vi "BASE-Main.vi"() -> ()   [LabVIEW 2017]
uses:
  <vilib>/Utility/error.llb/DialogType.ctl
  55ed0eea-cd20-493f-8468-85b8c1a0a0c0.vi
panel:
  out "Status Number":i32
  out "Status":i32(ring)=1 items=["Stopped"=1, "StartPending"=2, "StopPending"=3, "Running"=4, "ContinuePending"=5, "PausePending"=6, "Paused"=7]
  in  "Modify SN":bool
  in  "PRINT":bool
  in  "Torque IO Status":bool
  in  "Ass IO Status":bool
  in  "Recipe":bool
  out "error out":errorcluster
  in  "Logout":bool
  in  "Stop":bool
  in  "Create Login":bool
  in  "Reports":bool
  in  "Start":bool
  out "Time":string
  out "Date":string
  in  "Login":bool
  # "KAPSE SONS ROBOTICS\n& AUTOMATION"
  # "RBC ORVM"
types:
  T1 = typedef "DialogType.ctl" = u16
  T2 = enum32{"Invalid", "Standard", "Closed", "Hidden", "Minimized", "Maximized"}
  T3 = enum8{"Enabled", "Disabled", "Disabled and Grayed Out"}
  T4 = enum32{"invalid app kind", "Development System", "Run Time System", "Student Edition", "Embedded LabVIEW", "Evaluation", "Custom"}
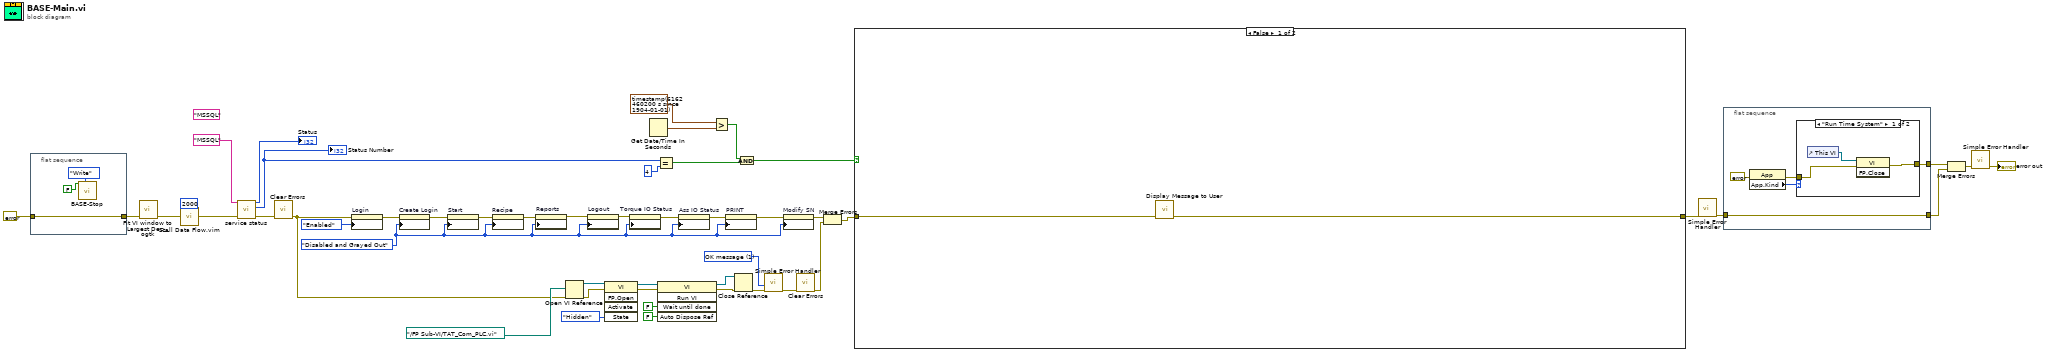
[diagram p0: block diagram]
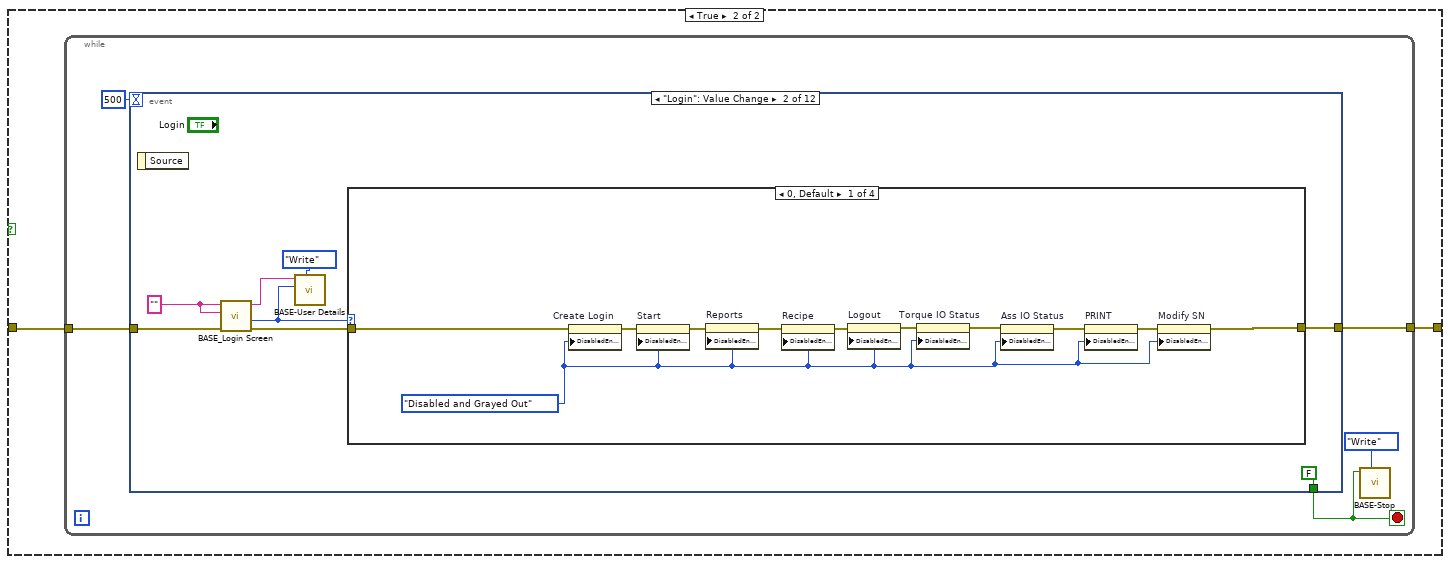
[diagram p3: hidden frame]
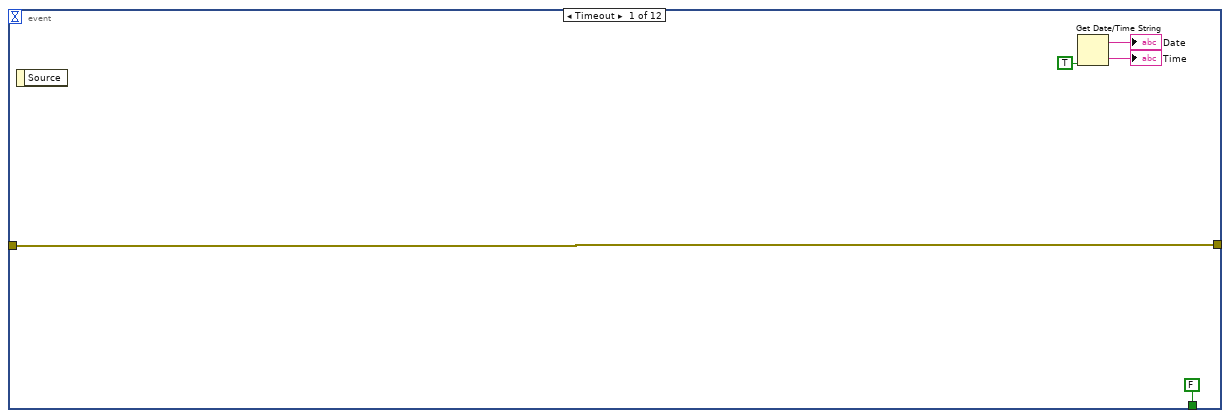
[diagram p4: hidden frame]
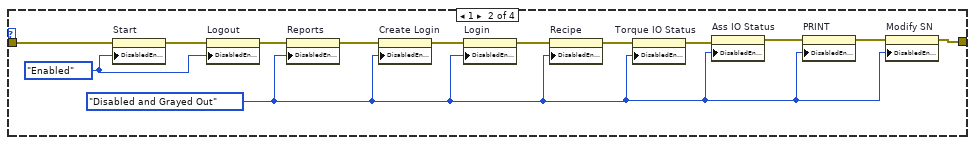
[diagram p5: hidden frame]
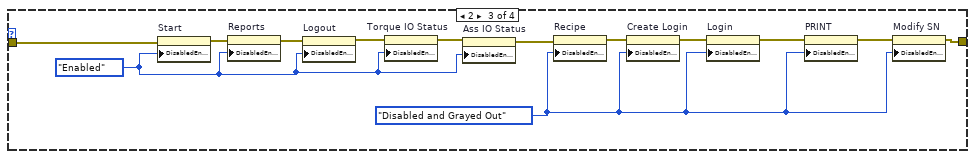
[diagram p6: hidden frame]
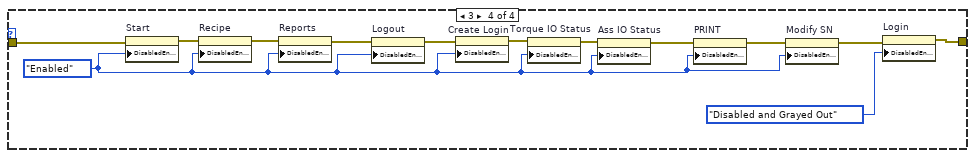
[diagram p7: hidden frame]
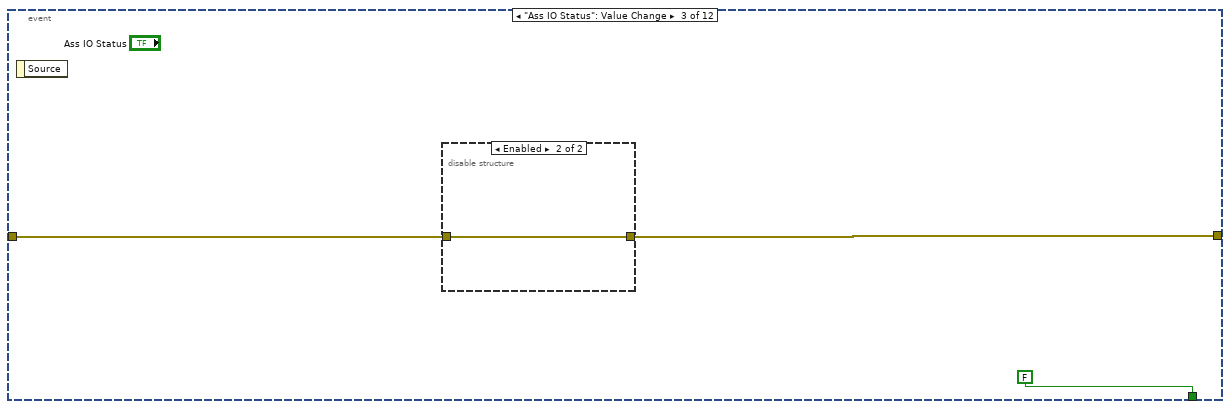
[diagram p8: hidden frame]
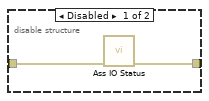
[diagram p9: hidden frame]
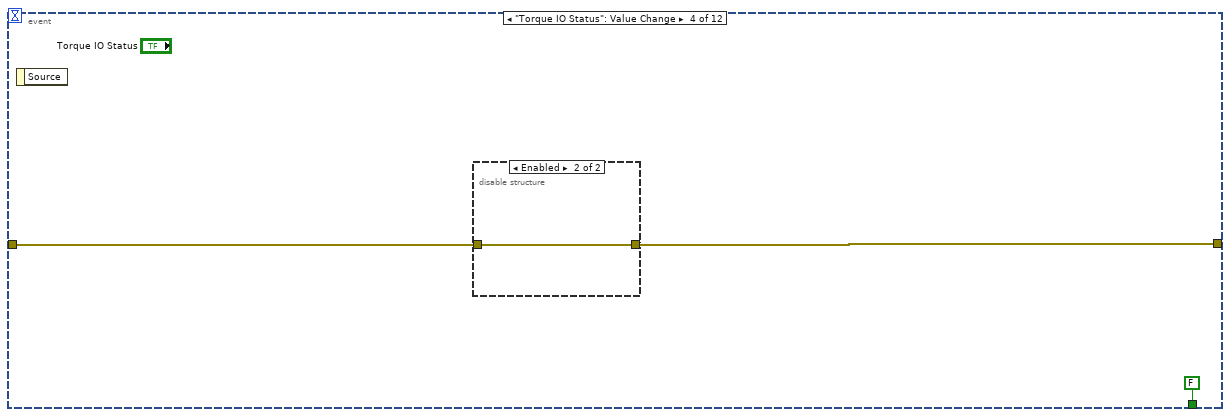
[diagram p10: hidden frame]
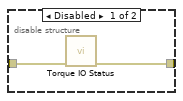
[diagram p11: hidden frame]
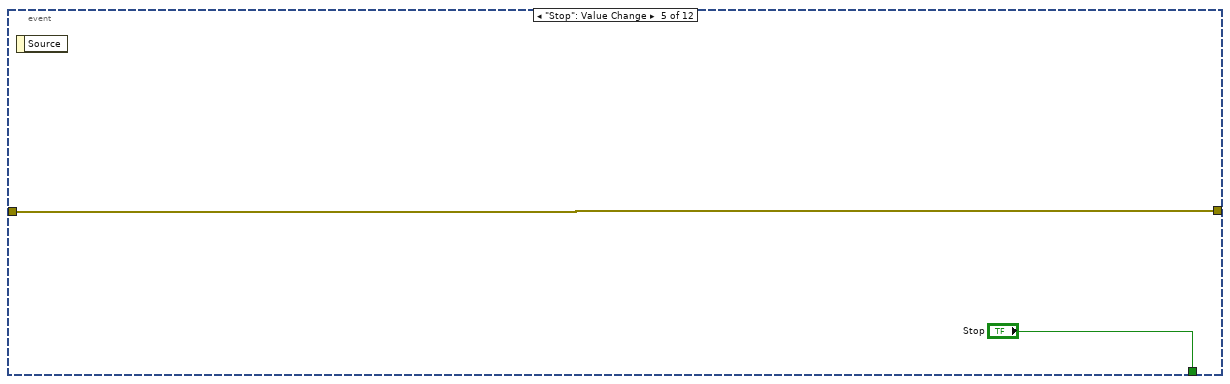
[diagram p12: hidden frame]
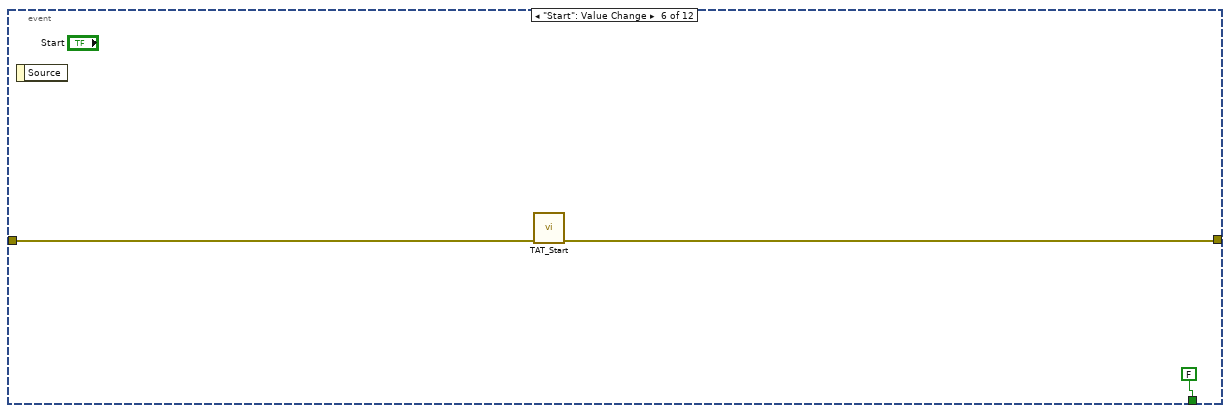
[diagram p13: hidden frame]
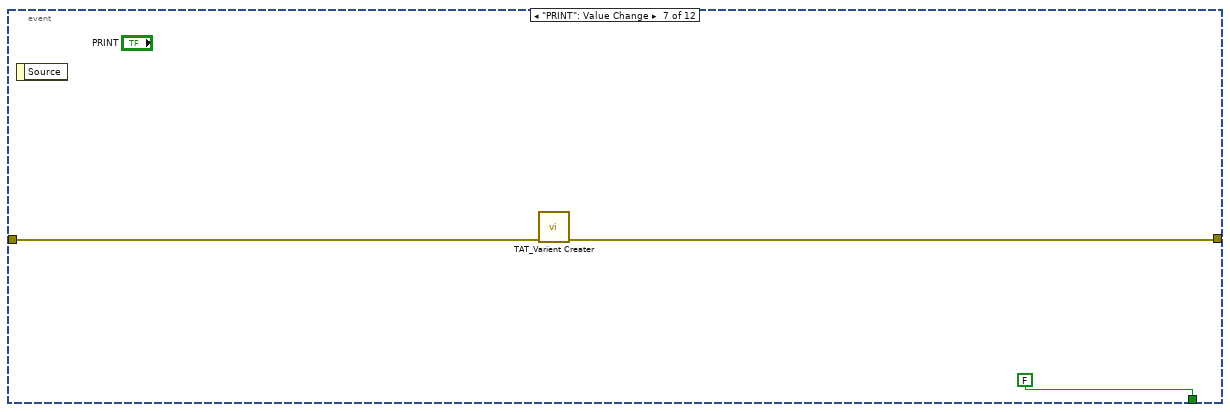
[diagram p14: hidden frame]
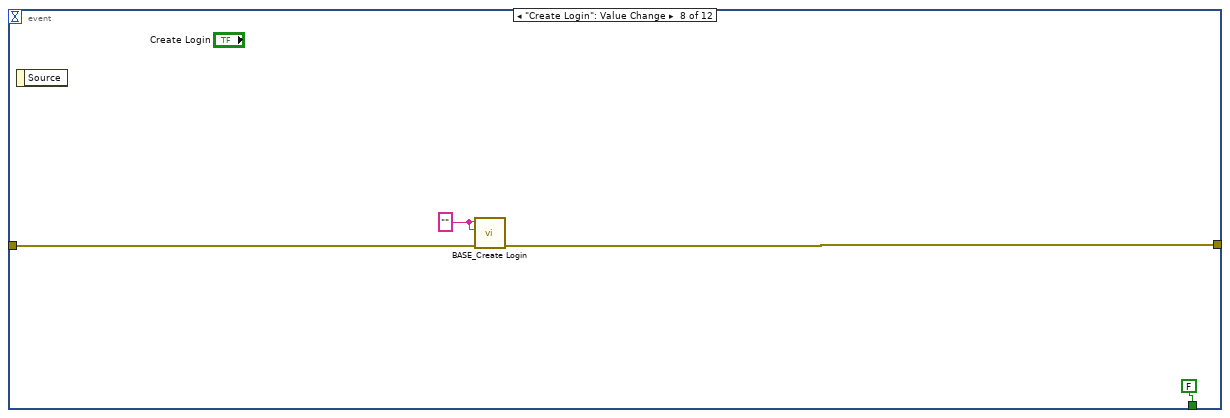
[diagram p15: hidden frame]
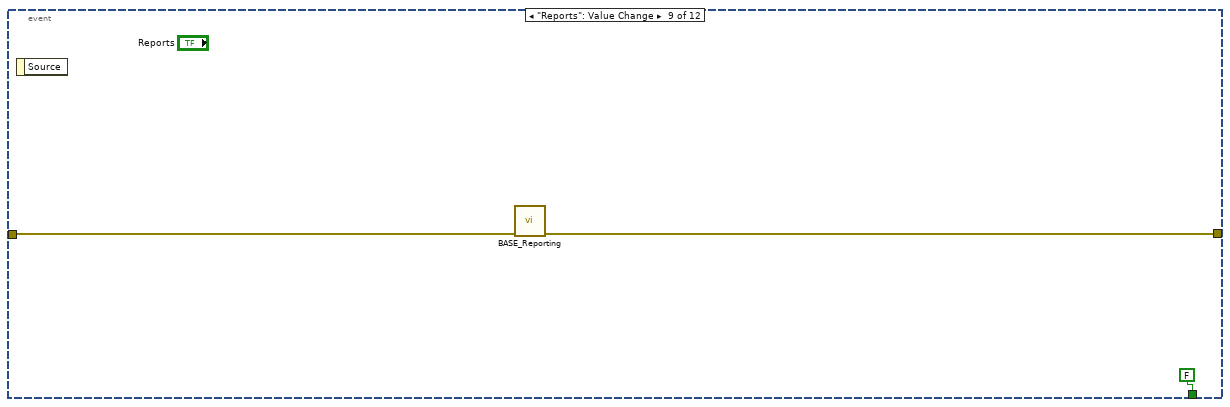
[diagram p16: hidden frame]
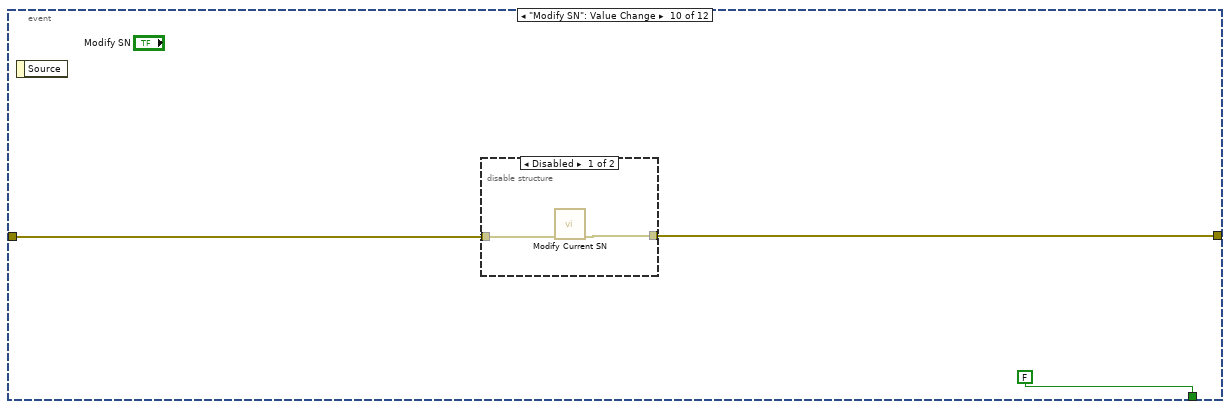
[diagram p17: hidden frame]
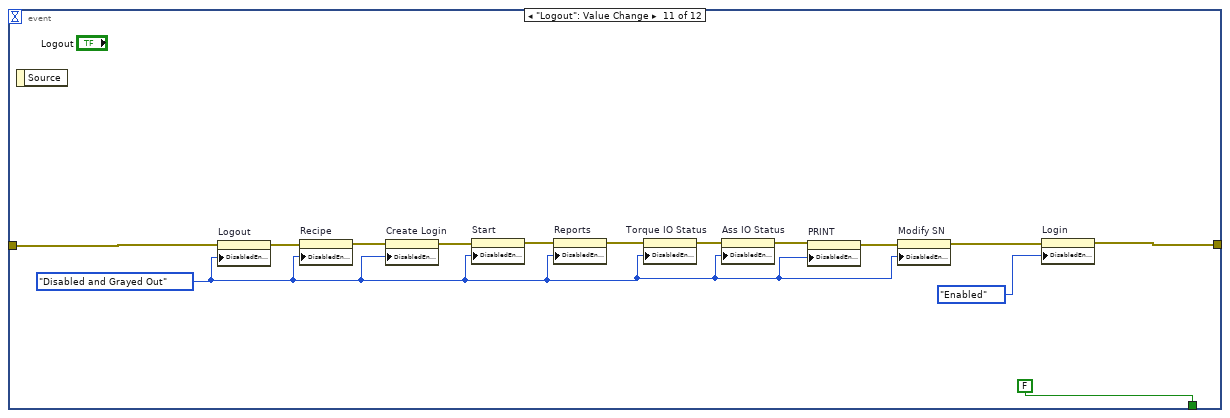
[diagram p19: hidden frame]
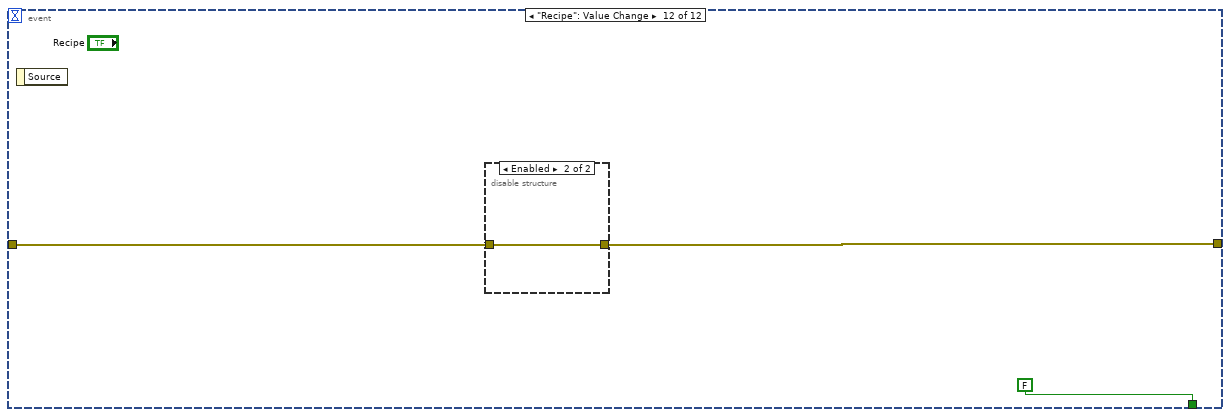
[diagram p20: hidden frame]
diagram:
  (unwired) "MSSQL" ("Service Name")
  w18 = T1 1 items=["no dialog", "OK message", "continue or stop message", "OK message + warnings", "continue/stop + warnings"] ("type of dialog (OK msg:1)")
  w33 = T3."Disabled and Grayed Out" ("Disabled")
  n1 = flat-sequence {
    tunnel: [w52] -> w32
    tunnel: errorcluster {"status"=FALSE, "code"=0, "source"=""} ("error constant") -> [w52]
    frame #0 {
      n2 = call "BASE-Stop.vi"("Enum"=enum16{"Read", "Write"}."Write", "Stop"=FALSE) -> ()  [unwired: 9 in, 1 out]
    }
  }
  n3 = call <userlib>:"Fit VI window to Largest Dec__ogtk.vi"("error in (no error)"=w32) -> ("error out"=w3:errorcluster)  [unwired: 5 in, 1 out]
  n4 = call "Stall Data Flow.vim"("value in"=w3, "milliseconds to wait"=u32 2000) -> ("value out"=w2:errorcluster)  [unwired: 1 out]
  n5 = call "service status.vi"("error in"=w2, "Service Name"="MSSQL") -> ("error out"=w10:errorcluster, "Status Number"=w12:i32, "Status"=→"Status":i32)  [unwired: 6 in, 1 out]
  "Status Number" <- w12
  n6 = call <vilib>:"Clear Errors.vi"("error in (no error)"=w10) -> ("error out"=w9:errorcluster)  [unwired: 5 in, 1 out]
  n7 = property on="Login" class="Bool"(error in=w9, "DisabledEnum"=T3."Enabled" ("Disabled")) -> (error out=w43:errorcluster)  [unwired: 1 in, 1 out]
  n8 = property on="Create Login" class="Bool"(error in=w43, "DisabledEnum"=w33) -> (error out=w48:errorcluster)  [unwired: 1 in, 1 out]
  n9 = property on="Start" class="Bool"(error in=w48, "DisabledEnum"=w33) -> (error out=w39:errorcluster)  [unwired: 1 in, 1 out]
  n10 = property on="Recipe" class="Bool"(error in=w39, "DisabledEnum"=w33) -> (error out=w38:errorcluster)  [unwired: 1 in, 1 out]
  n11 = property on="Reports" class="Bool"(error in=w38, "DisabledEnum"=w33) -> (error out=w41:errorcluster)  [unwired: 1 in, 1 out]
  n12 = Open VI Reference(vi path=path "../FP Sub-VI/TAT_Com_PLC.vi", error in (no error)=w9) -> (vi reference=w28:refnum<vi>, error out=w29:errorcluster)  [unwired: 4 in]
  n13 = property on="Logout" class="Bool"(error in=w41, "DisabledEnum"=w33) -> (error out=w37:errorcluster)  [unwired: 1 in, 1 out]
  n14 = invoke class="VI" method="FP.Open"(reference=w28, error in=w29, "State"=T2."Hidden") -> (reference out=w31:refnum<vi>, error out=w30:errorcluster)  [unwired: 2 in, 3 out]
  n15 = property on="Torque IO Status" class="Bool"(error in=w37, "DisabledEnum"=w33) -> (error out=w36:errorcluster)  [unwired: 1 in, 1 out]
  n16 = Get Date/Time In Seconds() -> (seconds since 1Jan1904=w5:timestamp)
  n17 = Equal?(x=w12, y=4) -> (x = y?=w8:bool)
  n18 = invoke class="VI" method="Run VI"(reference=w31, error in=w30, "Wait until done"=FALSE ("Wait Until Done"), "Auto Dispose Ref"=FALSE ("Auto Dispose Reference")) -> (reference out=w27:refnum<vi>, error out=w26:errorcluster)  [unwired: 1 in, 3 out]
  n19 = property on="Ass IO Status" class="Bool"(error in=w36, "DisabledEnum"=w33) -> (error out=w35:errorcluster)  [unwired: 1 in, 1 out]
  n20 = Greater?(x=timestamp(6162460200 s since 1904-01-01), y=w5) -> (0:w4:bool)
  n21 = property on="PRINT" class="Bool"(error in=w35, "DisabledEnum"=w33) -> (error out=w34:errorcluster)  [unwired: 1 in, 1 out]
  n22 = Close Reference(reference=w27, error in (no error)=w26) -> (error out=w19:errorcluster)
  n23 = And(x=w4, y=w8) -> (x .and. y?=w7:bool)
  n24 = call <vilib>:"Simple Error Handler.vi"("type of dialog (OK msg:1)"=w18, "error in (no error)"=w19) -> ("error out"=w17:errorcluster)  [unwired: 3 in, 4 out]
  n25 = property on="Modify SN" class="Bool"(error in=w34, "DisabledEnum"=w33) -> (error out=w21:errorcluster)  [unwired: 1 in, 1 out]
  n26 = call <vilib>:"Clear Errors.vi"("error in (no error)"=w17) -> ("error out"=w16:errorcluster)  [unwired: 5 in, 1 out]
  n27 = Merge Errors(w21, w16) -> (w22:errorcluster)
  n28 = case shown="False" w7 {
    tunnel: w22 -> [w54 w56]
    tunnel: [w53 w55] -> w49
    frame False {
      n29 = call "Display Message to User"("error in (no error)"=w54) -> ("error out"=w53:errorcluster)  [unwired: 9 in, 1 out]
    }
    frame True {
      n30 = while {
        tunnel: w56 -> [w60]
        tunnel: [w59] -> w55
        stop <- w57 stop-if-true
        n31 = event shown="[1] \"Login\": Value Change" {
          selector: _ -> [_ _ _ _ _ _ _ _ _ _ _ _]
          dyn-events: _ -> [_ _ _ _ _ _ _ _ _ _ _ _]
          timeout: 500 -> [_ _ _ _ _ _ _ _ _ _ _ _]
          tunnel: w60 -> [w64 w74 w127 w132 w137 w140 w143 w148 w150 w154 w167 w173]
          tunnel: [w64 w72 w126 w131 w137 w139 w142 w147 w149 w153 w168 w172] -> w59
          tunnel: [FALSE ("Stop") FALSE ("Stop") FALSE ("Stop") FALSE ("Stop") "Stop" FALSE ("Stop") FALSE ("Stop") FALSE ("Stop") FALSE ("Stop") FALSE ("Stop") FALSE ("Stop") FALSE ("Stop")] -> w57
          event Timeout {
            n32 = event-data() -> ()  [unwired: 1 in, 1 out]
            n33 = Get Date/Time String(want seconds? (F)=TRUE) -> (date string=→"Date":string, time string=→"Time":string)  [unwired: 2 in]
          }
          event "Login": Value Change {
            w69 = "" ("User Name")
            n34 = event-data() -> ()  [unwired: 1 in, 1 out]
            n35 = call "BASE_Login Screen.vi"("Error In"=w74, "Password"=w69, "User Name"=w69) -> ("error out"=w73:errorcluster, "Level"=w67:i32, "User Name Out"=w70:string)  [unwired: 5 in, 1 out]
            n36 = call "BASE-User Details.vi"("Enum"=enum16{"Read", "Write"}."Write", "Level In"=w67, "User Name In"=w70) -> ()  [unwired: 7 in, 2 out]
            n37 = case shown="0, Default" w67 {
              tunnel: w73 -> [w83 w98 w111 w124]
              tunnel: [w76 w87 w100 w123] -> w72
              frame 0, Default {
                w75 = T3."Disabled and Grayed Out" ("Disabled")
                n38 = property on="Create Login" class="Bool"(error in=w83, "DisabledEnum"=w75) -> (error out=w85:errorcluster)  [unwired: 1 in, 1 out]
                n39 = property on="Start" class="Bool"(error in=w85, "DisabledEnum"=w75) -> (error out=w84:errorcluster)  [unwired: 1 in, 1 out]
                n40 = property on="Reports" class="Bool"(error in=w84, "DisabledEnum"=w75) -> (error out=w82:errorcluster)  [unwired: 1 in, 1 out]
                n41 = property on="Recipe" class="Bool"(error in=w82, "DisabledEnum"=w75) -> (error out=w81:errorcluster)  [unwired: 1 in, 1 out]
                n42 = property on="Logout" class="Bool"(error in=w81, "DisabledEnum"=w75) -> (error out=w80:errorcluster)  [unwired: 1 in, 1 out]
                n43 = property on="Torque IO Status" class="Bool"(error in=w80, "DisabledEnum"=w75) -> (error out=w79:errorcluster)  [unwired: 1 in, 1 out]
                n44 = property on="Ass IO Status" class="Bool"(error in=w79, "DisabledEnum"=w75) -> (error out=w78:errorcluster)  [unwired: 1 in, 1 out]
                n45 = property on="PRINT" class="Bool"(error in=w78, "DisabledEnum"=w75) -> (error out=w77:errorcluster)  [unwired: 1 in, 1 out]
                n46 = property on="Modify SN" class="Bool"(error in=w77, "DisabledEnum"=w75) -> (error out=w76:errorcluster)  [unwired: 1 in, 1 out]
              }
              frame 1 {
                w86 = T3."Disabled and Grayed Out" ("Disabled")
                w94 = T3."Enabled" ("Disabled")
                n47 = property on="Start" class="Bool"(error in=w98, "DisabledEnum"=w94) -> (error out=w93:errorcluster)  [unwired: 1 in, 1 out]
                n48 = property on="Logout" class="Bool"(error in=w93, "DisabledEnum"=w94) -> (error out=w96:errorcluster)  [unwired: 1 in, 1 out]
                n49 = property on="Reports" class="Bool"(error in=w96, "DisabledEnum"=w86) -> (error out=w97:errorcluster)  [unwired: 1 in, 1 out]
                n50 = property on="Create Login" class="Bool"(error in=w97, "DisabledEnum"=w86) -> (error out=w95:errorcluster)  [unwired: 1 in, 1 out]
                n51 = property on="Login" class="Bool"(error in=w95, "DisabledEnum"=w86) -> (error out=w92:errorcluster)  [unwired: 1 in, 1 out]
                n52 = property on="Recipe" class="Bool"(error in=w92, "DisabledEnum"=w86) -> (error out=w90:errorcluster)  [unwired: 1 in, 1 out]
                n53 = property on="Torque IO Status" class="Bool"(error in=w90, "DisabledEnum"=w86) -> (error out=w91:errorcluster)  [unwired: 1 in, 1 out]
                n54 = property on="Ass IO Status" class="Bool"(error in=w91, "DisabledEnum"=w86) -> (error out=w89:errorcluster)  [unwired: 1 in, 1 out]
                n55 = property on="PRINT" class="Bool"(error in=w89, "DisabledEnum"=w86) -> (error out=w88:errorcluster)  [unwired: 1 in, 1 out]
                n56 = property on="Modify SN" class="Bool"(error in=w88, "DisabledEnum"=w86) -> (error out=w87:errorcluster)  [unwired: 1 in, 1 out]
              }
              frame 2 {
                w99 = T3."Disabled and Grayed Out" ("Disabled")
                w103 = T3."Enabled" ("Disabled")
                n57 = property on="Start" class="Bool"(error in=w111, "DisabledEnum"=w103) -> (error out=w108:errorcluster)  [unwired: 1 in, 1 out]
                n58 = property on="Reports" class="Bool"(error in=w108, "DisabledEnum"=w103) -> (error out=w110:errorcluster)  [unwired: 1 in, 1 out]
                n59 = property on="Logout" class="Bool"(error in=w110, "DisabledEnum"=w103) -> (error out=w105:errorcluster)  [unwired: 1 in, 1 out]
                n60 = property on="Torque IO Status" class="Bool"(error in=w105, "DisabledEnum"=w103) -> (error out=w106:errorcluster)  [unwired: 1 in, 1 out]
                n61 = property on="Ass IO Status" class="Bool"(error in=w106, "DisabledEnum"=w103) -> (error out=w104:errorcluster)  [unwired: 1 in, 1 out]
                n62 = property on="Recipe" class="Bool"(error in=w104, "DisabledEnum"=w99) -> (error out=w107:errorcluster)  [unwired: 1 in, 1 out]
                n63 = property on="Create Login" class="Bool"(error in=w107, "DisabledEnum"=w99) -> (error out=w109:errorcluster)  [unwired: 1 in, 1 out]
                n64 = property on="Login" class="Bool"(error in=w109, "DisabledEnum"=w99) -> (error out=w102:errorcluster)  [unwired: 1 in, 1 out]
                n65 = property on="PRINT" class="Bool"(error in=w102, "DisabledEnum"=w99) -> (error out=w101:errorcluster)  [unwired: 1 in, 1 out]
                n66 = property on="Modify SN" class="Bool"(error in=w101, "DisabledEnum"=w99) -> (error out=w100:errorcluster)  [unwired: 1 in, 1 out]
              }
              frame 3 {
                w112 = T3."Enabled" ("Disabled")
                n67 = property on="Start" class="Bool"(error in=w124, "DisabledEnum"=w112) -> (error out=w119:errorcluster)  [unwired: 1 in, 1 out]
                n68 = property on="Recipe" class="Bool"(error in=w119, "DisabledEnum"=w112) -> (error out=w118:errorcluster)  [unwired: 1 in, 1 out]
                n69 = property on="Reports" class="Bool"(error in=w118, "DisabledEnum"=w112) -> (error out=w121:errorcluster)  [unwired: 1 in, 1 out]
                n70 = property on="Logout" class="Bool"(error in=w121, "DisabledEnum"=w112) -> (error out=w120:errorcluster)  [unwired: 1 in, 1 out]
                n71 = property on="Create Login" class="Bool"(error in=w120, "DisabledEnum"=w112) -> (error out=w117:errorcluster)  [unwired: 1 in, 1 out]
                n72 = property on="Torque IO Status" class="Bool"(error in=w117, "DisabledEnum"=w112) -> (error out=w116:errorcluster)  [unwired: 1 in, 1 out]
                n73 = property on="Ass IO Status" class="Bool"(error in=w116, "DisabledEnum"=w112) -> (error out=w115:errorcluster)  [unwired: 1 in, 1 out]
                n74 = property on="PRINT" class="Bool"(error in=w115, "DisabledEnum"=w112) -> (error out=w114:errorcluster)  [unwired: 1 in, 1 out]
                n75 = property on="Modify SN" class="Bool"(error in=w114, "DisabledEnum"=w112) -> (error out=w113:errorcluster)  [unwired: 1 in, 1 out]
                n76 = property on="Login" class="Bool"(error in=w113, "DisabledEnum"=T3."Disabled and Grayed Out" ("Disabled")) -> (error out=w123:errorcluster)  [unwired: 1 in, 1 out]
              }
            }
          }
          event "Ass IO Status": Value Change {
            n77 = event-data() -> ()  [unwired: 1 in, 1 out]
            n78 = disable-structure shown="Enabled" {
              disable-tunnel: w127 -> [w129 w130]
              disable-tunnel: [w128 w130] -> w126
              frame Disabled {
                n79 = call "Ass IO Status.vi"("error in (no error)"=w129) -> ("error out"=w128:errorcluster)  [unwired: 10 in]
              }
              frame Enabled {
              }
            }
          }
          event "Torque IO Status": Value Change {
            n80 = event-data() -> ()  [unwired: 1 in, 1 out]
            n81 = disable-structure shown="Enabled" {
              disable-tunnel: w132 -> [w135 w136]
              disable-tunnel: [w134 w136] -> w131
              frame Disabled {
                n82 = call "Torque IO Status.vi"("error in (no error)"=w135) -> ("error out"=w134:errorcluster)  [unwired: 10 in]
              }
              frame Enabled {
              }
            }
          }
          event "Stop": Value Change {
            n83 = event-data() -> ()  [unwired: 1 in, 1 out]
          }
          event "Start": Value Change {
            n84 = event-data() -> ()  [unwired: 1 in, 1 out]
            n85 = call "TAT_Start.vi"("error In"=w140) -> ("error out"=w139:errorcluster)  [unwired: 10 in]
          }
          event "PRINT": Value Change {
            n86 = event-data() -> ()  [unwired: 1 in, 1 out]
            n87 = call "TAT_Varient Creater.vi"("error in (no error)"=w143) -> ("error out"=w142:errorcluster)  [unwired: 10 in]
          }
          event "Create Login": Value Change {
            w146 = "" ("User Name")
            n88 = event-data() -> ()  [unwired: 1 in, 1 out]
            n89 = call "BASE_Create Login.vi"("Error In"=w148, "Password"=w146, "User Name"=w146) -> ("error out"=w147:errorcluster)  [unwired: 6 in]
          }
          event "Reports": Value Change {
            n90 = event-data() -> ()  [unwired: 1 in, 1 out]
            n91 = call "BASE_Reporting.vi"("error in (no error)"=w150) -> ("error out"=w149:errorcluster)  [unwired: 10 in]
          }
          event "Modify SN": Value Change {
            n92 = event-data() -> ()  [unwired: 1 in, 1 out]
            n93 = disable-structure shown="Disabled" {
              disable-tunnel: w154 -> [w156 _]
              disable-tunnel: [w155 _] -> w153
              frame Disabled {
                n94 = call "Modify Current SN.vi"("error in (no error)"=w156) -> ("error out"=w155:errorcluster)  [unwired: 10 in]
              }
              frame Enabled {
              }
            }
          }
          event "Logout": Value Change {
            w157 = T3."Disabled and Grayed Out" ("Disabled")
            n95 = event-data() -> ()  [unwired: 1 in, 1 out]
            n96 = property on="Logout" class="Bool"(error in=w167, "DisabledEnum"=w157) -> (error out=w165:errorcluster)  [unwired: 1 in, 1 out]
            n97 = property on="Recipe" class="Bool"(error in=w165, "DisabledEnum"=w157) -> (error out=w164:errorcluster)  [unwired: 1 in, 1 out]
            n98 = property on="Create Login" class="Bool"(error in=w164, "DisabledEnum"=w157) -> (error out=w170:errorcluster)  [unwired: 1 in, 1 out]
            n99 = property on="Start" class="Bool"(error in=w170, "DisabledEnum"=w157) -> (error out=w169:errorcluster)  [unwired: 1 in, 1 out]
            n100 = property on="Reports" class="Bool"(error in=w169, "DisabledEnum"=w157) -> (error out=w162:errorcluster)  [unwired: 1 in, 1 out]
            n101 = property on="Torque IO Status" class="Bool"(error in=w162, "DisabledEnum"=w157) -> (error out=w163:errorcluster)  [unwired: 1 in, 1 out]
            n102 = property on="Ass IO Status" class="Bool"(error in=w163, "DisabledEnum"=w157) -> (error out=w160:errorcluster)  [unwired: 1 in, 1 out]
            n103 = property on="PRINT" class="Bool"(error in=w160, "DisabledEnum"=w157) -> (error out=w159:errorcluster)  [unwired: 1 in, 1 out]
            n104 = property on="Modify SN" class="Bool"(error in=w159, "DisabledEnum"=w157) -> (error out=w158:errorcluster)  [unwired: 1 in, 1 out]
            n105 = property on="Login" class="Bool"(error in=w158, "DisabledEnum"=T3."Enabled" ("Disabled")) -> (error out=w168:errorcluster)  [unwired: 1 in, 1 out]
          }
          event "Recipe": Value Change {
            n106 = event-data() -> ()  [unwired: 1 in, 1 out]
            n107 = disable-structure shown="Enabled" {
              disable-tunnel: w173 -> [w175 w176]
              disable-tunnel: [w174 w176] -> w172
              frame Disabled {
                n108 = call "TAT-Create Reciepe.vi"("Error In"=w175) -> ("error out"=w174:errorcluster)  [unwired: 10 in]
              }
              frame Enabled {
              }
            }
          }
        }
        n109 = call "BASE-Stop.vi"("Enum"=enum16{"Read", "Write"}."Write", "Stop"=w57) -> ()  [unwired: 9 in, 1 out]
      }
    }
  }
  n110 = call <vilib>:"Simple Error Handler.vi"("error in (no error)"=w49) -> ("error out"=w44:errorcluster)  [unwired: 4 in, 4 out]
  n111 = flat-sequence {
    tunnel: [w178] -> w47
    tunnel: [w177] -> w45
    tunnel: w44 -> [w177]
    frame #0 {
      n112 = property class="App"(error in=errorcluster {"status"=FALSE, "code"=0, "source"=""} ("error in (no error)")) -> (error out=w180:errorcluster, "App.Kind"=w181:T4)  [unwired: 1 in, 1 out]
      n113 = case shown="\"Run Time System\"" w181 {
        tunnel: w180 -> [w183 w185]
        tunnel: [w182 w185] -> w178
        frame "Run Time System" {
          n114 = control-ref of="This VI"() -> (w184:refnum<vi>)
          n115 = invoke class="VI" method="FP.Close"(reference=w184, error in=w183) -> (error out=w182:errorcluster)  [unwired: 1 in, 2 out]
        }
        frame "Development System", Default {
        }
      }
    }
  }
  n116 = Merge Errors(w47, w45) -> (w46:errorcluster)
  n117 = call <vilib>:"Simple Error Handler.vi"("error in (no error)"=w46) -> ("error out"=→"error out":errorcluster)  [unwired: 4 in, 4 out]
